vi "Method Dialog_Setup Show Options.vi"(6 "Properties for Tree In":T1(array[cluster])=[{"Label"="a", "Tag"="a", "Property Type"=enum."Base", "Indent"=0, "Can Read?"=TRUE, "Can Write?"=TRUE, "Is Read?"=FALSE, "Is Write?"=TRUE, "Inactive Parent?"=FALSE, "Unwired?"=FALSE}, {"Label"="b", "Tag"="b", "Property Type"=enum."Scripting", "Indent"=0, "Can Read?"=TRUE, "Can Write?"=FALSE, "Is Read?"=FALSE, "Is Write?"=FALSE, "Inactive Parent?"=FALSE, "Unwired?"=FALSE}, {"Label"="c", "Tag"="c", "Property Type"=enum."Base", "Indent"=0, "Can Read?"=TRUE, "Can Write?"=TRUE, "Is Read?"=FALSE, "Is Write?"=FALSE, "Inactive Parent?"=FALSE, "Unwired?"=FALSE}, {"Label"="d", "Tag"="d", "Property Type"=enum."Private", "Indent"=0, "Can Read?"=TRUE, "Can Write?"=FALSE, "Is Read?"=FALSE, "Is Write?"=FALSE, "Inactive Parent?"=FALSE, "Unwired?"=FALSE}, {"Label"="E", "Tag"="E", "Property Type"=enum."Base", "Indent"=0, "Can Read?"=TRUE, "Can Write?"=TRUE, "Is Read?"=FALSE, "Is Write?"=TRUE, "Inactive Parent?"=FALSE, "Unwired?"=FALSE}, {"Label"="f", "Tag"="f", "Property Type"=enum."Base", "Indent"=0, "Can Read?"=TRUE, "Can Write?"=FALSE, "Is Read?"=FALSE, "Is Write?"=FALSE, "Inactive Parent?"=FALSE, "Unwired?"=FALSE}], 11 "Cluster in":refnum<vi>) -> ()   [LabVIEW 2023]
doc: "Show/hide option booleans for \n\n--Show script/schow private\n--Select unwired termainls (remove items action)"
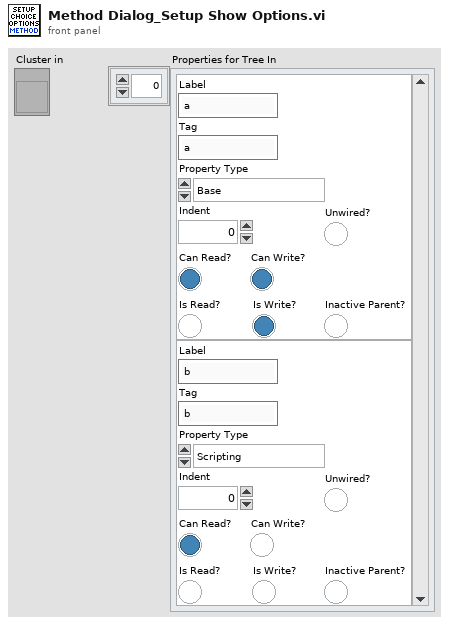
[diagram p1: front panel]
types:
  T1 = cluster{"Label":string, "Tag":string, "Property Type":enum16{"Unknown", "Base", "Scripting", "Private", "Deprecated", "None", "Divider"}, "Indent":u16, "Can Read?":bool, "Can Write?":bool, "Is Read?":bool, "Is Write?":bool, "Inactive Parent?":bool, "Unwired?":bool}[]
  T2 = enum8{"Enabled", "Disabled", "Disabled and Grayed Out"}
  T3 = enum16{"Unknown", "Base", "Scripting", "Private", "Deprecated", "None", "Divider"}
  T4 = cluster{"Show Scripting":bool, "Show Private":bool}
  T5 = enum8{"Enabled", "Disabled", "Disabled and Grayed Out"}[]
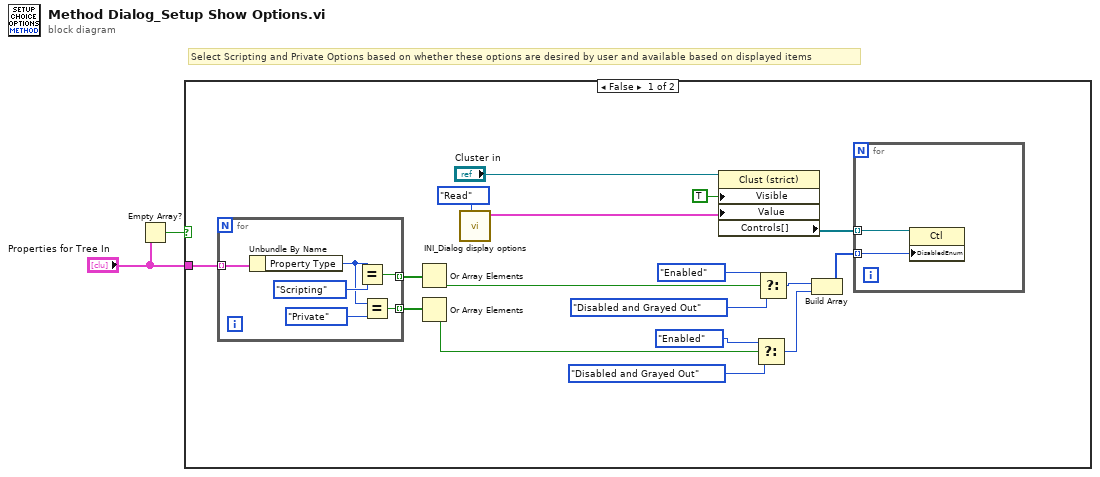
[diagram p0: block diagram]
diagram:
  # "Select Scripting and Private Options based on whether these options are desired by user and available based on displayed items"
  n1 = Empty Array?(array="Properties for Tree In") -> (empty?=w2:bool)
  n2 = case shown="False" w2 {
    tunnel: "Properties for Tree In" -> [w18 _]
    frame False {
      n3 = for {
        tunnel: w18 -> [w27] mode=indexing
        tunnel: [w25] -> w17 mode=indexing
        tunnel: [w22] -> w16 mode=indexing
        n4 = Unbundle By Name(w27) -> ("Property Type"=w24:T3)
        n5 = Equal?(x=w24, y=T3."Scripting" ("Property Type")) -> (x = y?=w25:bool)
        n6 = Equal?(x=w24, y=T3."Private" ("Property Type")) -> (x = y?=w22:bool)
      }
      n7 = Or Array Elements(Boolean array=w17) -> (logical OR=w15:bool)
      n8 = Or Array Elements(Boolean array=w16) -> (logical OR=w14:bool)
      n9 = call "INI_Dialog display options.vi"("File Action"=enum16{"Read", "Write"}."Read") -> ("Display Options Out"=w13:T4)  [unwired: 10 in]
      n10 = property class="Clust (strict)"(reference="Cluster in", "Visible"=TRUE, "Value"=w13) -> ("Controls[]"=w10:refnum<vi>[])  [unwired: 1 in, 2 out]
      n11 = Select(t=T2."Enabled" ("Disabled"), s=w14, f=T2."Disabled and Grayed Out" ("Disabled")) -> (s? t:f=w5:T2)
      n12 = Select(t=T2."Enabled" ("Disabled"), s=w15, f=T2."Disabled and Grayed Out" ("Disabled")) -> (s? t:f=w6:T2)
      n13 = Build Array(w6, w5) -> (w3:T5)
      n14 = for {
        tunnel: w10 -> [w21] mode=indexing
        tunnel: w3 -> [w20] mode=indexing
        n15 = property class="Ctl"(reference=w21, "DisabledEnum"=w20) -> ()  [unwired: 1 in, 2 out]
      }
    }
    frame True {
    }
  }
